vi "loadDatabase.vi"(8 "error in (no error)":errorcluster, 11 "deviceDataBase in":refnum<class "deviceDataBase.lvclass">) -> (0 "error out":errorcluster, 1 "total":dbl format="%_9g", 3 "deviceDataBase out":refnum<class "deviceDataBase.lvclass">)   [LabVIEW 2009, in "Tools.lvlib" / "DatabaseHelpers.lvlib" / "deviceDataBase.lvclass"]
doc: "DeviceDataBase Load.\n\nLoad the Device Database into this object for use by everyone who need access to it.\nAccess is provided by a functional Global."
uses:
  deviceDataBase.lvclass
  Filing/FileSystem/FileSystem.lvclass
  deviceDataBase.lvclass/deviceDataBase.ctl
  Database Objects/device/device.lvclass
  Database Objects/DeviceArray/DeviceArray.lvclass
  Database Objects/ChannelArray/ChannelArray.lvclass
  NativeXML/NativeXML.lvclass
panel:
  out "labels":string[](array[string])
  out "Array 2":T1(array[ring])
  out "read":dbl format="%_9g"
  out "open":dbl format="%_9g"
  out "Array":string[](array[string])
  out "channelNames":string[](array[string])
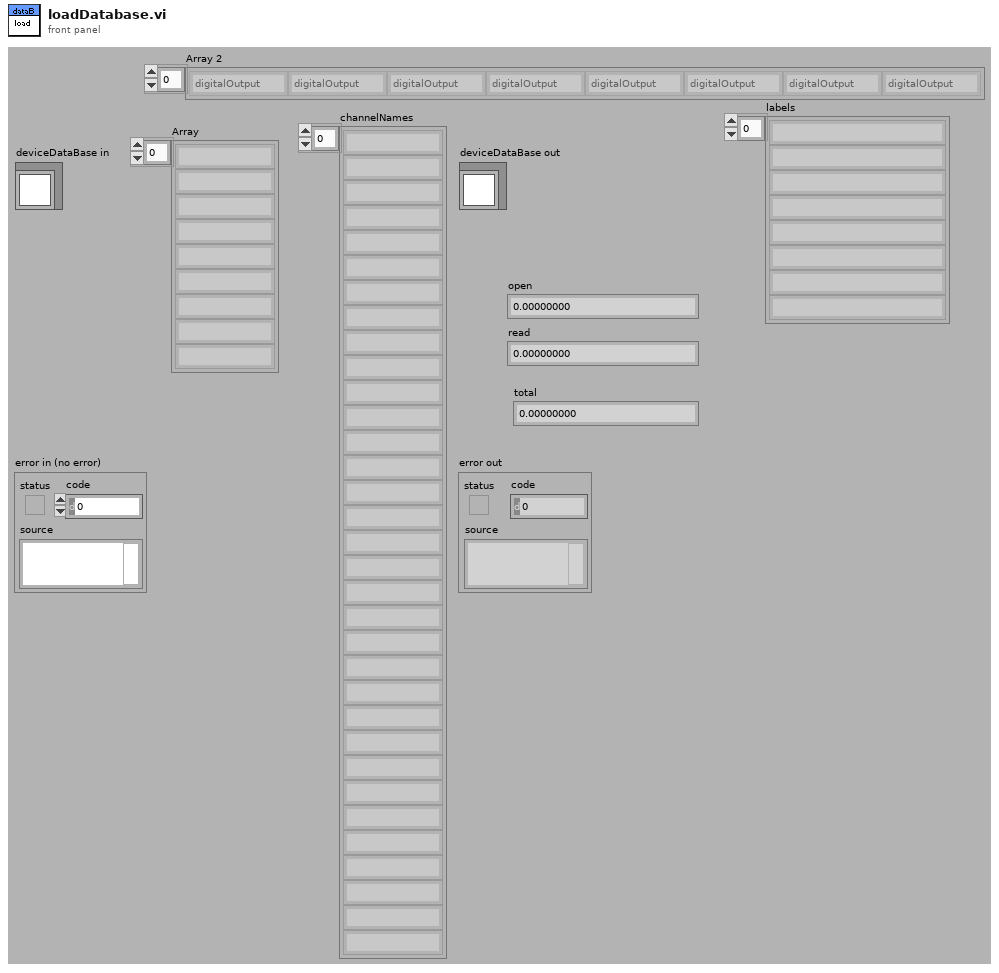
[diagram p1: front panel]
types:
  T1 = enum16{"digitalOutput", "digitalInput", "analogOutput", "analogInput", "rfOutput", "ethernetSupply"}[]
  T2 = enum16{"digitalOutput", "digitalInput", "analogOutput", "analogInput", "rfOutput", "ethernetSupply"}
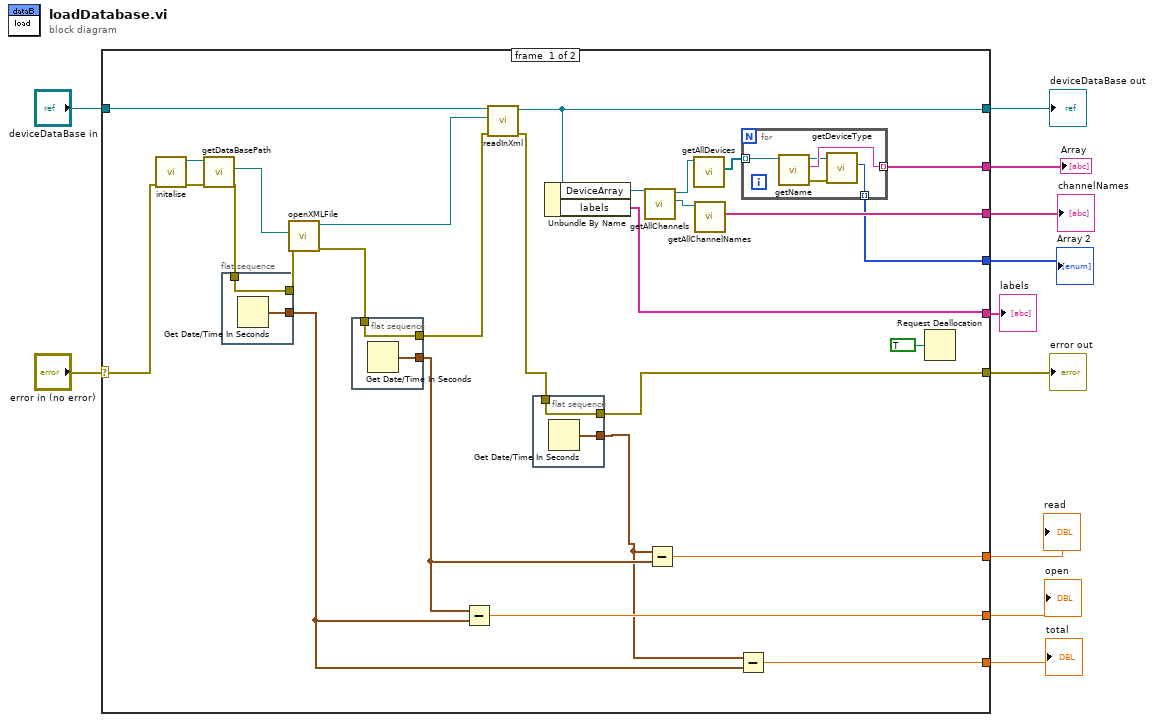
[diagram p0: block diagram]
diagram:
  n1 = case shown="No Error" "error in (no error)" {
    selector: "error in (no error)" -> [w37 w52]
    tunnel: [w20 w52] -> w10
    tunnel: [w35 w51] -> w8
    tunnel: "deviceDataBase in" -> [w36 w51]
    tunnel: [w32 _] -> w7
    tunnel: [w29 _] -> w6
    tunnel: [w28 _] -> w5
    tunnel: [w19 _] -> w4
    tunnel: [w17 _] -> w3
    tunnel: [w14 _] -> w2
    tunnel: [w12 _] -> w1
    frame #0 {
      n2 = call "initalise.vi"("error in (no error)"=w37) -> ("error out"=w39:errorcluster, "FileSystem out"=w38:refnum<class "FileSystem.lvclass">)  [unwired: 9 in]
      n3 = call-dynamic "getDataBasePath.vi"("error in (no error)"=w39, "FileSystem.lvclass in"=w38) -> ("error out"=w25:errorcluster, "DataBasePath"=w27:path)  [unwired: 7 in, 1 out]
      n4 = flat-sequence {
        tunnel: w25 -> [w45]
        tunnel: [w45] -> w24
        tunnel: [w44] -> w15
        frame #0 {
          n5 = Get Date/Time In Seconds() -> (seconds since 1Jan1904=w44:timestamp)
        }
      }
      n6 = call "openXMLFile.vi"("error in (no error)"=w24, "Path"=w27) -> ("error out"=w23:errorcluster, "NativeXML out"=w26:refnum<class "NativeXML.lvclass">)  [unwired: 8 in]
      n7 = flat-sequence {
        tunnel: w23 -> [w43]
        tunnel: [w43] -> w22
        tunnel: [w42] -> w18
        frame #0 {
          n8 = Get Date/Time In Seconds() -> (seconds since 1Jan1904=w42:timestamp)
        }
      }
      n9 = Subtract(x=w18, y=w15) -> (x-y=w19:dbl)
      n10 = call "readInXml.vi"("error in (no error)"=w22, "NativeXML out"=w26, "deviceDataBase in"=w36) -> ("error out"=w21:errorcluster, "deviceDataBase out"=w35:refnum<class "deviceDataBase.lvclass">)  [unwired: 7 in]
      n11 = flat-sequence {
        tunnel: w21 -> [w41]
        tunnel: [w41] -> w20
        tunnel: [w40] -> w16
        frame #0 {
          n12 = Get Date/Time In Seconds() -> (seconds since 1Jan1904=w40:timestamp)
        }
      }
      n13 = Unbundle By Name(w35) -> ("DeviceArray"=w34:refnum<class "DeviceArray.lvclass">, "labels"=w12:string[])
      n14 = call "getAllChannels.vi"("DeviceArray in"=w34) -> ("ChannelArray.lvclass"=w33:refnum<class "ChannelArray.lvclass">, "DeviceArray out"=w31:refnum<class "DeviceArray.lvclass">)  [unwired: 8 in, 1 out]
      n15 = Subtract(x=w16, y=w18) -> (x-y=w17:dbl)
      n16 = call "getAllDevices.vi"("DeviceArray.lvclass in"=w31) -> ("deviceArray"=w30:refnum<class "device.lvclass">[])  [unwired: 8 in, 2 out]
      n17 = call "getAllChannelNames.vi"("ChannelArray in"=w33) -> ("channelNames"=w32:string[])  [unwired: 8 in, 2 out]
      n18 = Subtract(x=w16, y=w15) -> (x-y=w14:dbl)
      n19 = for {
        tunnel: w30 -> [w50] mode=indexing
        tunnel: [w49] -> w29 mode=indexing
        tunnel: [w46] -> w28 mode=indexing
        n20 = call "getName.vi"("device.lvclass in"=w50) -> ("error out"=w47:errorcluster, "name"=w49:string, "device.lvclass out"=w48:refnum<class "device.lvclass">)  [unwired: 8 in]
        n21 = call-dynamic "getDeviceType.vi"("error in (no error)"=w47, "device.lvclass in"=w48) -> ("type"=w46:T2)  [unwired: 7 in, 2 out]
      }
      n22 = Request Deallocation(TRUE ("flag")) -> ()
    }
    frame #1 {
    }
  }
  "error out" <- w10
  "deviceDataBase out" <- w8
  "channelNames" <- w7
  "Array" <- w6
  "open" <- w4
  "read" <- w3
  "total" <- w2
  "Array 2" <- w5
  "labels" <- w1
